vi "Create Persistent Unified.vi"(9 "Persistent Core Actor":refnum<class "Actor.lvclass">, 10 "Persistent Decorator Actors":refnum<class "Actor.lvclass">[](array[class])) -> (1 "Persistent Unified Msgs":T1, 2 "Persistent Unified Actor":refnum<class "Actor.lvclass">)   [LabVIEW 2025, in "jettl.lvlib"]
uses:
  jettl.lvlib
  Actor/Actor.lvclass
  Msgs.ctl
  Msg/Msg.lvclass
  Base Actor/Base Actor.lvlib
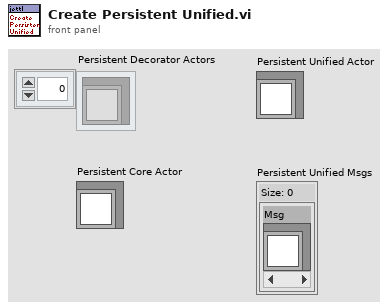
[diagram p1: front panel]
types:
  T1 = typedef "jettl.lvlib/Msgs.ctl" = set{refnum<class "Msg.lvclass">}
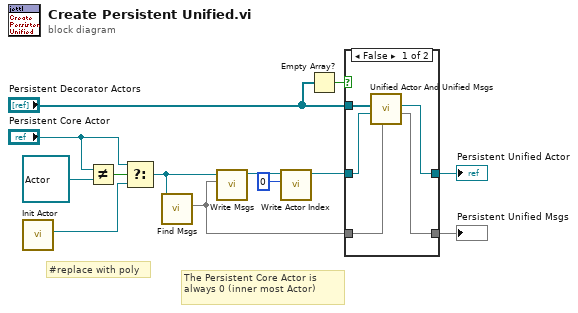
[diagram p0: block diagram]
diagram:
  # "The Persistent Core Actor is always 0 (inner most Actor)"
  # "#replace with poly"
  n1 = call "Init Actor.vi"() -> ("Actor"=w11:refnum<class "Actor.lvclass">)  [unwired: 11 in]
  n2 = Not Equal?(x="Persistent Core Actor", y=refnum<class "Actor.lvclass"> refnum ("Persistent Core Actor")) -> (x != y?=w12:bool)
  n3 = Select(t="Persistent Core Actor", s=w12, f=w11) -> (s? t:f=w10:refnum<class "Actor.lvclass">)
  n4 = call-dynamic "Find Msgs.vi"("Actor in"=w10) -> ("Msgs"=w6:T1)  [unwired: 10 in]
  n5 = call-dynamic "Write Msgs.vi"("Msgs"=w6, "Actor in"=w10) -> ("Actor out"=w3:refnum<class "Actor.lvclass">)  [unwired: 9 in]
  n6 = call-dynamic "Write Actor Index.vi"("Actor Index"=0, "Actor in"=w3) -> ("Actor out"=w2:refnum<class "Actor.lvclass">)  [unwired: 9 in]
  n7 = Empty Array?(array="Persistent Decorator Actors") -> (empty?=w8:bool)
  n8 = case shown="False" w8 {
    tunnel: w2 -> [w17 w20]
    tunnel: [w14 w20] -> w5
    tunnel: "Persistent Decorator Actors" -> [w18 _]
    tunnel: w6 -> [w16 w19]
    tunnel: [w15 w19] -> w4
    frame False {
      n9 = call "Unified Actor And Unified Msgs.vi"("Current Persistent Unified Msgs"=w16, "Current Persistent Unified Actor"=w17, "Decorator Actors"=w18) -> ("Unified Msgs"=w15:T1, "Unified Actor"=w14:refnum<class "Actor.lvclass">)  [unwired: 7 in]
    }
    frame True {
    }
  }
  "Persistent Unified Actor" <- w5
  "Persistent Unified Msgs" <- w4
